vi "create_arb_waveform.vi"(0 "Waveform Parameters":T1={"Constant"=1.0, "Nickname"="", "Conversion"=enum."B Field Grad (G/cm)"}, 1 "Sample rate":dbl, 2 "Time":dbl) -> (3 "Samples to Write":dbl, 4 "dt":dbl, 5 "Tau (exponential)":dbl, 6 "output waveform":waveform(dbl)(graph))   [LabVIEW 2015]
uses:
  6733_Red_MOT/6733_voltage_conversions.ctl
  Controls/6713/6713_static_waveform_item.ctl
panel:
  out "Numeric":i32
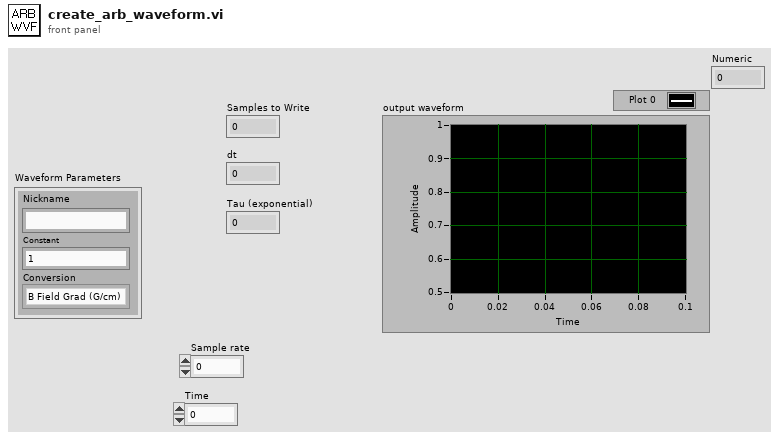
[diagram p1: front panel]
types:
  T1 = typedef "6713_static_waveform_item.ctl" = cluster{"Constant":dbl, "Nickname":string, "Conversion":T2}
  T2 = typedef "6733_voltage_conversions.ctl" = enum16{"B Field Grad (G/cm)", "Red MOT Center Freq (MHz)", "Red Dither Pk(kHz)", "Red Power (mW)", "Volts"}
  T3 = cluster{"Waveform Parameters":T1, "Time":dbl, "Sample rate":dbl}
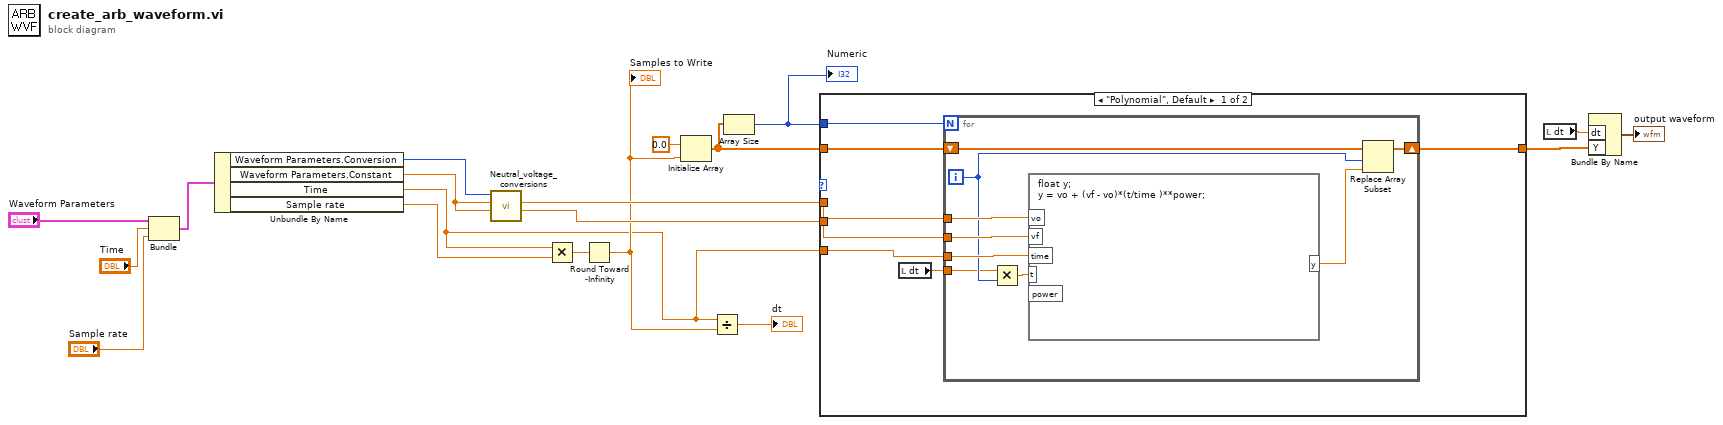
[diagram p0: block diagram]
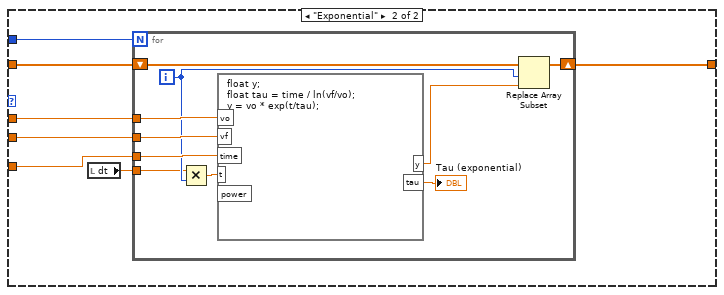
[diagram p2: hidden frame]
diagram:
  n1 = Bundle("Waveform Parameters"="Waveform Parameters", "Time"="Time", "Sample rate"="Sample rate") -> (w8:T3)  [unwired: 1 in]
  n2 = Unbundle By Name(w8) -> ("Waveform Parameters.Conversion"=w2:T2, "Waveform Parameters.Constant"=w1:dbl, "Time"=w3:dbl, "Sample rate"=w5:dbl)
  n3 = call "Neutral_voltage_conversions.vi"("Final Value"=w1, "Initial value"=w1, "Conversion"=w2) -> ("Final Voltage"=w6:dbl, "Initial voltage"=w7:dbl)  [unwired: 7 in]
  n4 = Multiply(x=w3, y=w5) -> (x*y=w12:dbl)
  n5 = Round Toward -Infinity(1:w12) -> (0:w4:dbl)
  "Samples to Write" <- w4
  n6 = Initialize Array(0.0 ("element"), w4) -> (w14:dbl[])
  n7 = Divide(x=w3, y=w4) -> (x/y=→"dt":dbl)
  n8 = Array Size(array=w14) -> (size(s)=w13:i32)
  "Numeric" <- w13
  n9 = case shown="\"Polynomial\", Default" {
    selector: _ -> [_ _]
    tunnel: w14 -> [w26 w42]
    tunnel: [w25 w41] -> w18
    tunnel: w7 -> [w24 w40]
    tunnel: w6 -> [w23 w39]
    tunnel: w3 -> [w22 w38]
    tunnel: w13 -> [w20 w36]
    frame "Polynomial", Default {
      n10 = local read "dt"() -> (w21:dbl)
      n11 = for {
        N: w20 -> [_]
        shift-right: [w34] -> w25
        shift-left: w26 -> [w35]
        tunnel: w24 -> [w33]
        tunnel: w23 -> [w32]
        tunnel: w22 -> [w31]
        tunnel: w21 -> [w28]
        i -> [w29]
        n12 = Multiply(x=w28, y=w29) -> (x*y=w30:dbl)
        n13 = formula code="float y;\ny = vo + (vf - vo)*(t/time )**power;"("vo"=w33, "vf"=w32, "time"=w31, "t"=w30) -> ("y"=w27:dbl)  [unwired: 1 in]
        n14 = Replace Array Subset(array=w35, new element=w27, index=w29) -> (w34:dbl[])
      }
    }
    frame "Exponential" {
      n15 = local read "dt"() -> (w37:dbl)
      n16 = for {
        N: w36 -> [_]
        shift-right: [w51] -> w41
        shift-left: w42 -> [w52]
        tunnel: w40 -> [w50]
        tunnel: w39 -> [w49]
        tunnel: w38 -> [w48]
        tunnel: w37 -> [w45]
        i -> [w46]
        n17 = Multiply(x=w45, y=w46) -> (x*y=w47:dbl)
        n18 = formula code="float y;\nfloat tau = time / ln(vf/vo);\ny = vo * exp(t/tau);"("vo"=w50, "vf"=w49, "time"=w48, "t"=w47) -> ("y"=w44:dbl, "tau"=→"Tau (exponential)":dbl)  [unwired: 1 in]
        n19 = Replace Array Subset(array=w52, new element=w44, index=w46) -> (w51:dbl[])
      }
    }
  }
  n20 = local read "dt"() -> (w16:dbl)
  n21 = Bundle By Name("dt"=w16, "Y"=w18) -> (→"output waveform":waveform(dbl))  [unwired: 1 in]
